vi "GetStabilizedPressureData.vi"(6 "Graph in":T1, 7 "WaitTime":i32, 8 "error in":errorcluster, 9 "SampleCount":i32, 10 "Variance/Mean Trigger":dbl, 11 "MinimalWaitTimems":u32) -> (0 "error out":errorcluster, 2 "Values":T1, 3 "StabilityAchieved":bool)   [LabVIEW 2012]
uses:
  GlobalVariables/AllowContinuousPressureAcquisition.vi
  GlobalVariables/IndexCaptor.vi
  GlobalVariables/IndexFlowmeter.vi
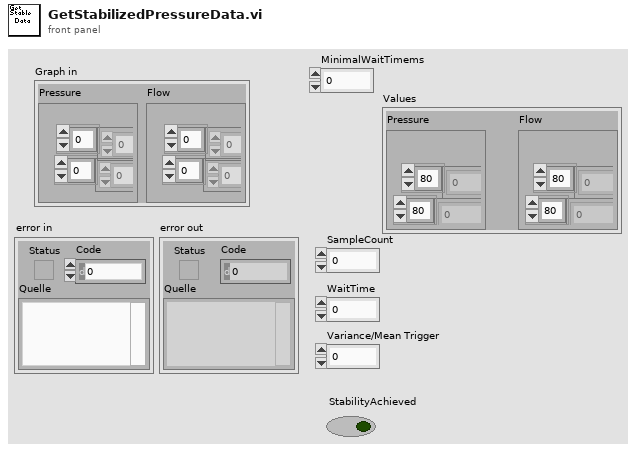
[diagram p1: front panel]
types:
  T1 = cluster{"Pressure":cluster{dbl[], dbl[]}, "Flow":cluster{dbl[], dbl[]}}
  T2 = cluster{"Values":cluster{dbl[], dbl[]}, "Values":cluster{dbl[], dbl[]}}
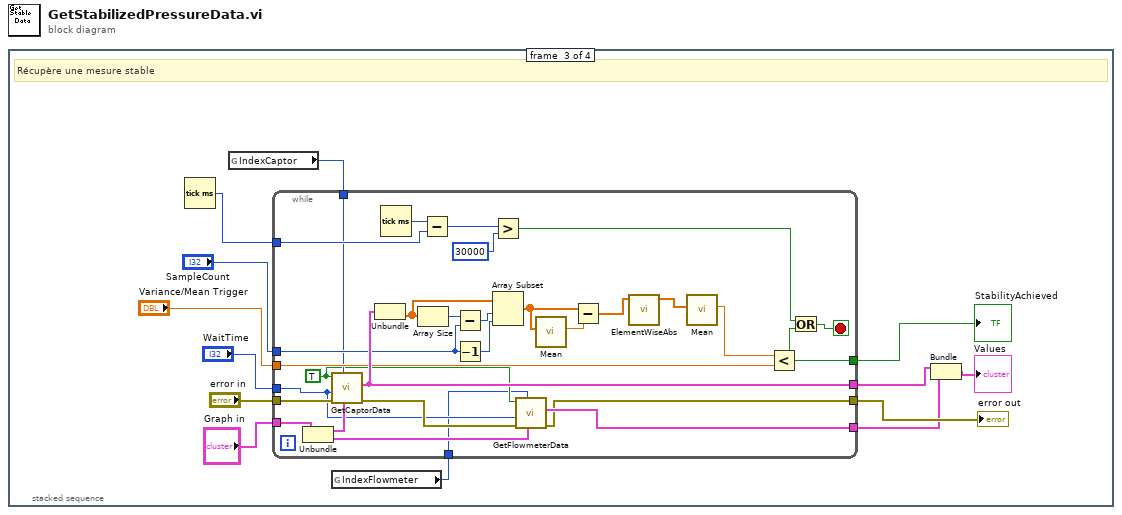
[diagram p0: block diagram]
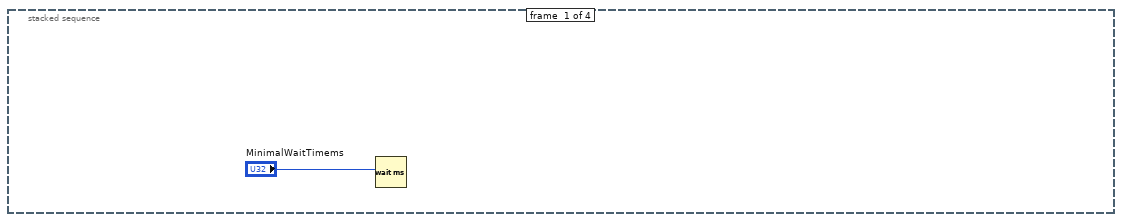
[diagram p2: hidden frame]
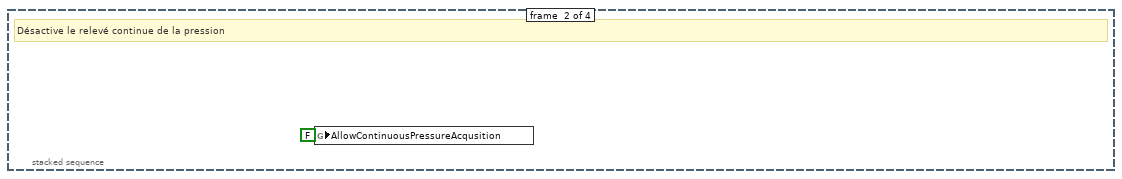
[diagram p3: hidden frame]
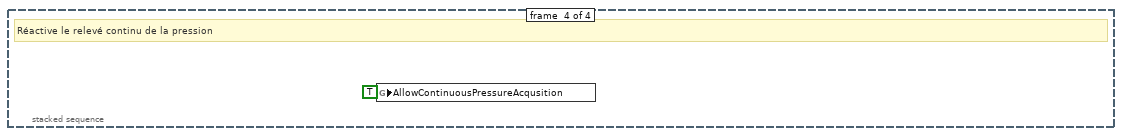
[diagram p4: hidden frame]
diagram:
  n1 = stacked-sequence {
    frame #0 {
      n2 = Wait (ms)(milliseconds to wait="MinimalWaitTimems") -> ()  [unwired: 1 out]
    }
    frame #1 {
      # "Désactive le relevé continue de la pression"
      n3 = global write "AllowContinuousPressureAcquisition.vi" "AllowContinuousPressureAcqusition"(FALSE) -> ()
    }
    frame #2 {
      # "Récupère une mesure stable"
      n4 = Tick Count (ms)() -> (millisecond timer value=w9:u32)
      n5 = global read "IndexCaptor.vi" "IndexCaptor"() -> (w4:i32)
      n6 = global read "IndexFlowmeter.vi" "IndexFlowmeter"() -> (w3:i32)
      n7 = while {
        tunnel: "error in" -> [w24]
        tunnel: [w19] -> w13
        tunnel: "Graph in" -> [w26]
        tunnel: [w42] -> w6
        tunnel: "SampleCount" -> [w39]
        tunnel: "Variance/Mean Trigger" -> [w41]
        tunnel: "WaitTime" -> [w18]
        tunnel: w9 -> [w32]
        tunnel: [w27] -> w8
        tunnel: [w22] -> w5
        tunnel: w4 -> [w23]
        tunnel: w3 -> [w16]
        stop <- w29 stop-if-true
        w17 = TRUE
        n8 = Unbundle(w26) -> ("Pressure"=w25:cluster{dbl[], dbl[]}, "Flow"=w21:cluster{dbl[], dbl[]})
        n9 = call "GetCaptorData.vi"("Graph in"=w25, "Index"=w23, "error in"=w24, "Length"=w18, "ON"=w17) -> ("error out"=w20:errorcluster, "Values"=w42:cluster{dbl[], dbl[]})  [unwired: 5 in]
        n10 = Unbundle(w42) -> (w45:dbl[])  [unwired: 1 out]
        n11 = Tick Count (ms)() -> (millisecond timer value=w33:u32)
        n12 = Array Size(array=w45) -> (size(s)=w44:i32)
        n13 = Subtract(x=w33, y=w32) -> (x-y=w31:u32)
        n14 = Subtract(x=w44, y=w39) -> (x-y=w43:i32)
        n15 = Decrement(x=w39) -> (x-1=w37:i32)
        n16 = Greater?(x=w31, y=u32 30000 ("x")) -> (0:w28:bool)
        n17 = Array Subset(array=w45, index=w43, length=w37) -> (w40:dbl[])
        n18 = call "GetFlowmeterData.vi"("Graph in"=w21, "Index"=w16, "error in"=w20, "Length"=w18, "ON"=w17) -> ("error out"=w19:errorcluster, "Values"=w22:cluster{dbl[], dbl[]})  [unwired: 5 in]
        n19 = call "Mean.vi"("Array"=w40) -> ("Mean"=w38:dbl)  [unwired: 10 in]
        n20 = Subtract(x=w40, y=w38) -> (x-y=w36:dbl[])
        n21 = call "ElementWiseAbs.vi"("Array [in]"=w36) -> ("Array[out]"=w35:dbl[])  [unwired: 10 in]
        n22 = call "Mean.vi"("Array"=w35) -> ("Mean"=w34:dbl)  [unwired: 10 in]
        n23 = Less?(x=w34, y=w41) -> (x < y?=w27:bool)
        n24 = Or(x=w28, y=w27) -> (x .or. y?=w29:bool)
      }
      "error out" <- w13
      "StabilityAchieved" <- w8
      n25 = Bundle("Values"=w6, "Values"=w5) -> (→"Values":T2)  [unwired: 1 in]
    }
    frame #3 {
      # "Réactive le relevé continu de la pression"
      n26 = global write "AllowContinuousPressureAcquisition.vi" "AllowContinuousPressureAcqusition"(TRUE) -> ()
    }
  }
